vi "Write Cal On.vi"(8 "error in (no error)":errorcluster, 10 "Cal On?":bool, 11 "Pressure Calibration Command in":refnum<class "Pressure Calibration Command.lvclass">) -> (0 "error out":errorcluster, 3 "Pressure Calibration Command out":refnum<class "Pressure Calibration Command.lvclass">)   [LabVIEW 2014, in "Pressure Calibration Command.lvclass"]
uses:
  Pressure Calibration Command.lvclass
  Pressure Calibration Command.lvclass/Pressure Calibration Command.ctl
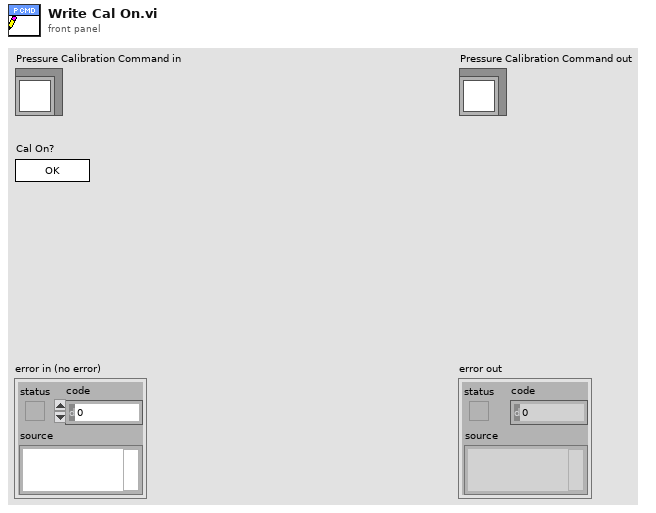
[diagram p1: front panel]
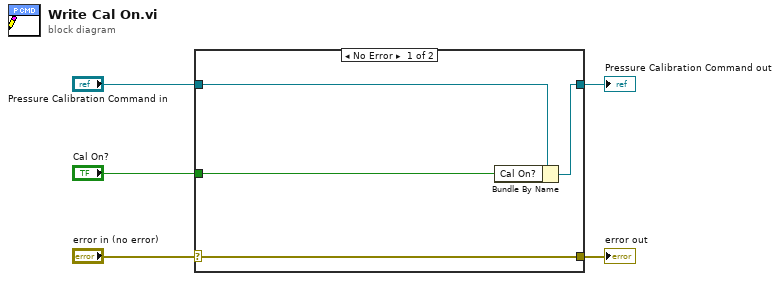
[diagram p0: block diagram]
diagram:
  n1 = case shown="No Error" "error in (no error)" {
    selector: "error in (no error)" -> [w9 w10]
    tunnel: [w9 w10] -> w4
    tunnel: [w7 w11] -> w2
    tunnel: "Pressure Calibration Command in" -> [w8 w11]
    tunnel: "Cal On?" -> [w6 _]
    frame No Error {
      n2 = Bundle By Name(cluster=w8, "Cal On?"=w6) -> (w7:refnum<class "Pressure Calibration Command.lvclass">)
    }
    frame Error {
    }
  }
  "error out" <- w4
  "Pressure Calibration Command out" <- w2
